vi "Hysteresis-CalculateCovariance.vi"(11 "Pictures":cluster{"Image 2":dbl[][], "Image 1":dbl[][]}) -> (3 "covariance":dbl)   [LabVIEW 2016]
uses:
  <vilib>/Analysis/baseanly.llb/Mean (DBL).vi
  <vilib>/Analysis/NI_AALBase.lvlib
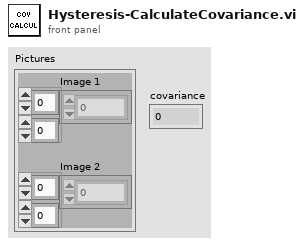
[diagram p1: front panel]
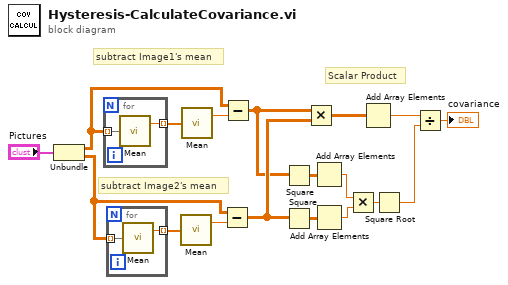
[diagram p0: block diagram]
diagram:
  # "Scalar Product"
  # "subtract Image2's mean"
  # "subtract Image1's mean"
  n1 = Unbundle("Pictures") -> ("Image 2"=w2:dbl[][], "Image 1"=w1:dbl[][])
  n2 = for {
    tunnel: w2 -> [w20] mode=indexing
    tunnel: [w19] -> w15 mode=indexing
    n3 = call-poly <vilib>:"Mean.vi"("X"=w20) -> ("mean"=w19:dbl)  [unwired: 1 out]
  }
  n4 = for {
    tunnel: w1 -> [w22] mode=indexing
    tunnel: [w21] -> w16 mode=indexing
    n5 = call-poly <vilib>:"Mean.vi"("X"=w22) -> ("mean"=w21:dbl)  [unwired: 1 out]
  }
  n6 = call-poly <vilib>:"Mean.vi"("X"=w16) -> ("mean"=w14:dbl)  [unwired: 1 out]
  n7 = call-poly <vilib>:"Mean.vi"("X"=w15) -> ("mean"=w13:dbl)  [unwired: 1 out]
  n8 = Subtract(x=w1, y=w14) -> (x-y=w18:dbl[][])
  n9 = Subtract(x=w2, y=w13) -> (x-y=w17:dbl[][])
  n10 = Square(x=w17) -> (x^2=w9:dbl[][])
  n11 = Square(x=w18) -> (x^2=w8:dbl[][])
  n12 = Multiply(x=w17, y=w18) -> (x*y=w4:dbl[][])
  n13 = Add Array Elements(numeric array=w9) -> (sum=w10:dbl)
  n14 = Add Array Elements(numeric array=w8) -> (sum=w11:dbl)
  n15 = Multiply(x=w10, y=w11) -> (x*y=w6:dbl)
  n16 = Add Array Elements(numeric array=w4) -> (sum=w5:dbl)
  n17 = Square Root(x=w6) -> (sqrt(x)=w7:dbl)
  n18 = Divide(x=w5, y=w7) -> (x/y=→"covariance":dbl)
